vi "Get Available Calculations Property.vi"(8 "error in (no error)":errorcluster, 11 "Device Item Ref":T1=18446744073709551615 format="%.0x") -> (0 "error in (no error) out":errorcluster, 2 "Available Calculations":string[](array[string]), 3 "Device Item Ref out":T1=18446744073709551615 format="%.0x")   [LabVIEW 2015, in "Waveform-Processing-Custom-Device System Explorer.lvlib"]
uses:
  Waveform-Processing-Custom-Device System Explorer.lvlib
  <vilib>/NI Veristand/Custom Device API/Custom Device Item Ref.ctl
  Shared/Constants.vi
  <vilib>/NI Veristand/Custom Device API/Get Item Property (String Array).vi
  <vilib>/NI VeriStand/Custom Device API/Custom Device API.lvlib
  Shared/Waveform-Processing-Custom-Device Shared.lvlib
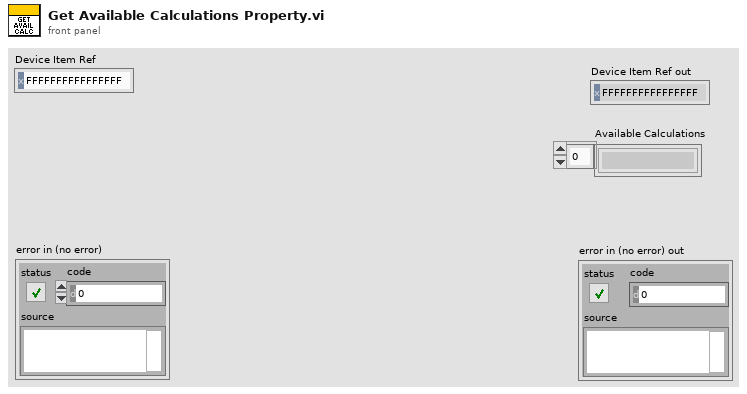
[diagram p1: front panel]
types:
  T1 = typedef "Custom Device API.lvlib/Custom Device Item Ref.ctl" = u64
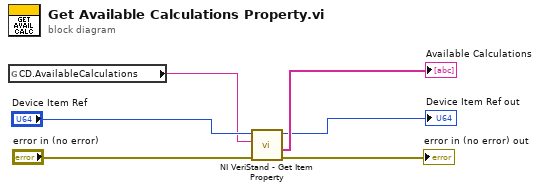
[diagram p0: block diagram]
diagram:
  n1 = global read "Constants.vi" "CD.AvailableCalculations"() -> (w4:string)
  n2 = call-poly <vilib>:"NI VeriStand - Get Item Property.vi"("error in (no error)"="error in (no error)", "Property Name"=w4, "Item Ref in"="Device Item Ref") -> ("error out"=→"error in (no error) out":errorcluster, "Value"=→"Available Calculations":string[], "Item Ref out"=→"Device Item Ref out":T1)  [unwired: 5 in, 1 out]
